vi "libssh2_channel_eof.vi"(8 "error in (no error)":errorcluster, 11 "channel":T1) -> (0 "error out":errorcluster, 2 "eof":bool)   [LabVIEW 2013, in "libssh2.lvlib"]
doc: "Checks if the remote host has sent an EOF status for the channel."
uses:
  libssh2.lvlib
  Channel Refnum.ctl
  Global Settings.vi
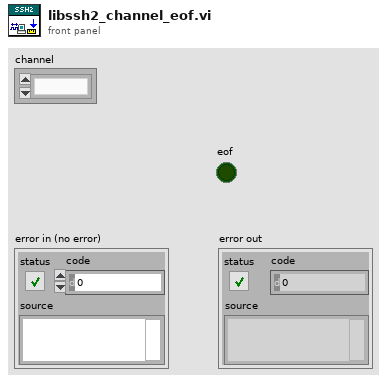
[diagram p1: front panel]
types:
  T1 = typedef "libssh2.lvlib/Channel Refnum.ctl" = refnum<k1>
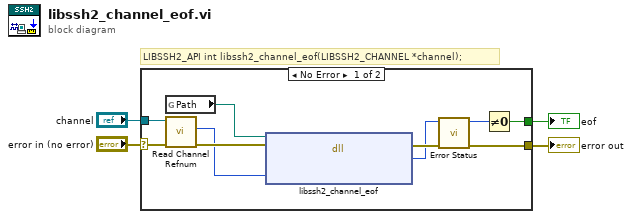
[diagram p0: block diagram]
diagram:
  # "LIBSSH2_API int libssh2_channel_eof(LIBSSH2_CHANNEL *channel);"
  n1 = case shown="No Error" "error in (no error)" {
    selector: "error in (no error)" -> [w10 w15]
    tunnel: [w8 w15] -> w4
    tunnel: "channel" -> [w11 _]
    tunnel: [w5 _] -> w1
    frame No Error {
      n2 = global read "Global Settings.vi" "Path"() -> (w9:path)
      n3 = call "Read Channel Refnum.vi"("error in (no error)"=w10, "channel"=w11) -> ("error out"=w13:errorcluster, "LIBSSH2_CHANNEL*"=w12:u64)  [unwired: 8 in]
      n4 = dll-call lib="C:/Users/pasca/source/repos/libssh2-labview/libssh2/libssh2**.*" fn="libssh2_channel_eof"(path in=w9, error in=w13, "channel"=w12) -> (error out=w14:errorcluster, "return value"=w7:i32)  [unwired: 2 in, 1 out]
      n5 = call "Error Status.vi"("error in (no error)"=w14, "return value"=w7) -> ("error out"=w8:errorcluster, "return value out"=w6:i32)  [unwired: 8 in]
      n6 = Not Equal To 0?(x=w6) -> (x != 0?=w5:bool)
    }
    frame Error {
    }
  }
  "error out" <- w4
  "eof" <- w1
